vi "Line break.vi"(8 "error in (no error)":errorcluster, 11 "Plain Text Report In":refnum<class "Plain Text Report.lvclass">) -> (0 "error out":errorcluster, 3 "Plain Text Report Out":refnum<class "Plain Text Report.lvclass">)   [LabVIEW 2020, in "Plain Text Report.lvclass"]
uses:
  Plain Text Report.lvclass
  Plain Text Report.lvclass/Plain Text Report.ctl
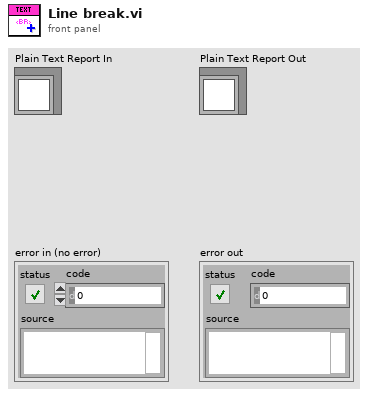
[diagram p1: front panel]
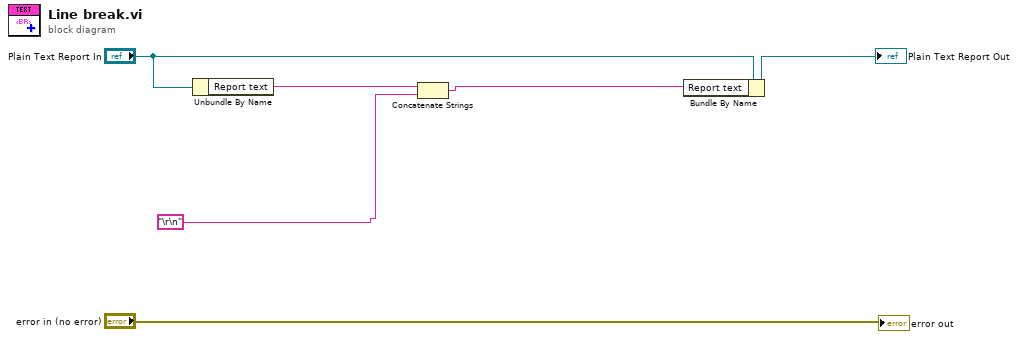
[diagram p0: block diagram]
diagram:
  n1 = Unbundle By Name("Plain Text Report In") -> ("Report text"=w3:string)
  n2 = Concatenate Strings(w3, "\r\n") -> (w2:string)
  n3 = Bundle By Name(cluster="Plain Text Report In", "Report text"=w2) -> (→"Plain Text Report Out":refnum<class "Plain Text Report.lvclass">)
  "error out" <- "error in (no error)"
